vi "TCP_Master_Global_ref.vi"(6 "Read:F/Wirte:T":bool, 8 "error in (no error) 2":errorcluster, 11 "ID IN":refnum<k5>) -> (0 "error out 2":errorcluster, 3 "ID OUT":refnum<k5>)   [LabVIEW 2022 SP3]
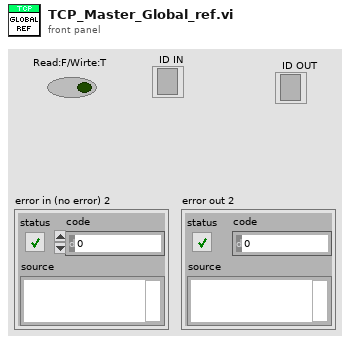
[diagram p1: front panel]
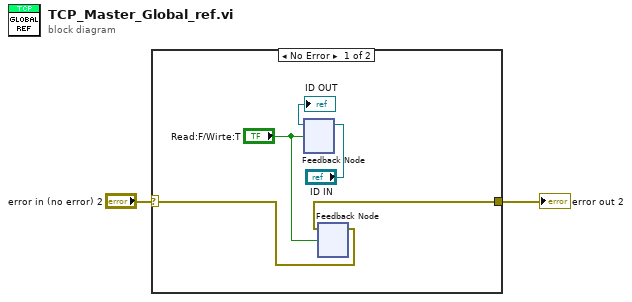
[diagram p0: block diagram]
diagram:
  n1 = case shown="No Error" "error in (no error) 2" {
    selector: "error in (no error) 2" -> [w5 w8]
    tunnel: [w4 w8] -> w1
    frame No Error {
      n2 = feedback-in #1("ID IN", "Read:F/Wirte:T") -> ()
      n3 = feedback #1() -> (→"ID OUT":refnum<k5>)  [unwired: 1 in]
      n4 = feedback #2() -> (w4:errorcluster)  [unwired: 1 in]
      n5 = feedback-in #2(w5, "Read:F/Wirte:T") -> ()
    }
    frame Error {
    }
  }
  "error out 2" <- w1
